vi "Delete Attribute Tree Data.vi"(7 "Tree ID":string, 8 "Error In":errorcluster, 10 "Attribute Name":string, 11 "Tree Manager":T1) -> (0 "Error Out":errorcluster, 1 "Attribute Value":refnum<class "Tree Data.lvclass">, 2 "Found?":bool, 3 "Tree Manager":T1)   [LabVIEW 2016, in "Tree Manager.lvclass"]
doc: "Delete a Tree Data typed attribute from the Tree and return it."
uses:
  Tree Manager.lvclass
  Typedefs/Session Handle.ctl
  Tree Data/Tree Data.lvclass
  Tree Manager.lvclass/Tree Manager.ctl
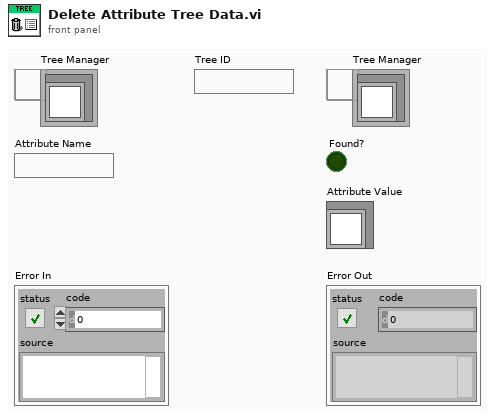
[diagram p1: front panel]
types:
  T1 = typedef "Tree Manager.lvclass/Session Handle.ctl" = refnum<data-value>
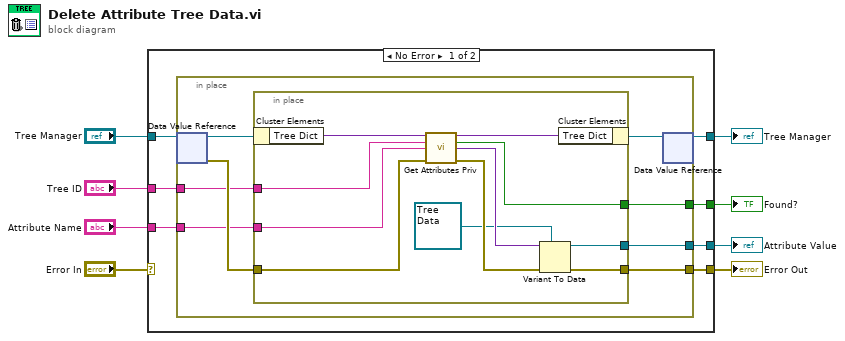
[diagram p0: block diagram]
diagram:
  n1 = case shown="No Error" "Error In" {
    selector: "Error In" -> [_ w35]
    tunnel: "Tree Manager" -> [w15 w36]
    tunnel: [w14 w36] -> w7
    tunnel: [w13 w35] -> w5
    tunnel: "Tree ID" -> [w12 _]
    tunnel: "Attribute Name" -> [w11 _]
    tunnel: [w10 _] -> w2
    tunnel: [w9 _] -> w1
    frame No Error {
      n2 = in-place {
        in-place-border: [w22] -> w13
        in-place-border: w12 -> [w19]
        in-place-border: w11 -> [w18]
        in-place-border: [w17] -> w10
        in-place-border: [w16] -> w9
        n3 = in-place-dvr #1(w15) -> (w23:refnum<class "Tree Manager.lvclass">, w20:errorcluster)
        n4 = in-place {
          in-place-border: [w28] -> w22
          in-place-border: w20 -> [w32]
          in-place-border: w19 -> [w31]
          in-place-border: w18 -> [w30]
          in-place-border: [w29] -> w17
          in-place-border: [w24] -> w16
          n5 = in-place-cluster #2(w23) -> ("Tree Dict"=w34:variant)
          n6 = call "Get Attributes Priv.vi"("Tree Dictionary In"=w34, "Unique ID"=w31, "Name"=w30, "error in"=w32) -> ("Tree Dictionary Out"=w33:variant, "Found?"=w29:bool, "Data"=w26:variant, "error out"=w27:errorcluster)  [unwired: 8 in]
          n7 = Variant To Data(error in=w27, type=refnum<class "Tree Data.lvclass"> refnum ("Tree Data.lvclass"), Variant=w26) -> (data=w24:refnum<class "Tree Data.lvclass">, error out=w28:errorcluster)
          n8 = in-place-cluster #2("Tree Dict"=w33) -> (w21:refnum<class "Tree Manager.lvclass">)
        }
        n9 = in-place-dvr #1(w21) -> (w14:T1)  [unwired: 1 out]
      }
    }
    frame Error {
    }
  }
  "Tree Manager" <- w7
  "Error Out" <- w5
  "Found?" <- w2
  "Attribute Value" <- w1
